vi "Actor Core.vi"(8 "error in":errorcluster, 11 "Interlock in":refnum<class "Interlock.lvclass">) -> (0 "error out":errorcluster, 3 "Actor out":refnum<class "Actor.lvclass">)   [LabVIEW 2015, in "Interlocks.lvlib" / "Interlock.lvclass"]
doc: "(<B>Filename</B>: Actor Framework.lvlib:Actor.lvclass:Actor Core.vi)\n\nReceives messages to the actor, reacts to them, and initiates any error handling that may shut the actor down.\n\nDescendant classes may override this VI to append parallel tasks for the actor to complete while it handles messages. Overrides use the Call Parent Method node."
uses:
  Interlock.lvclass
  <vilib>/ActorFramework/Actor/Actor.lvclass
  <vilib>/ActorFramework/Actor/Actor.lvclass/Actor.ctl
  <vilib>/ActorFramework/Message Enqueuer/Message Enqueuer.lvclass/Message Enqueuer.ctl
  <vilib>/ActorFramework/Message Enqueuer/Enqueue.vi
  <vilib>/ActorFramework/Message Enqueuer/Init from Existing Queue.vi
  <vilib>/ActorFramework/Message Priority Queue/Priority Enqueue.vi
  Interlock Messages/Invoke IL Action Msg/Invoke IL Action Msg.lvclass
  <vilib>/ActorFramework/Message Enqueuer/Message Enqueuer.lvclass
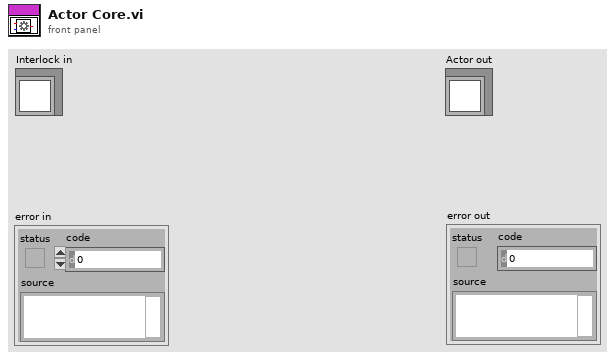
[diagram p1: front panel]
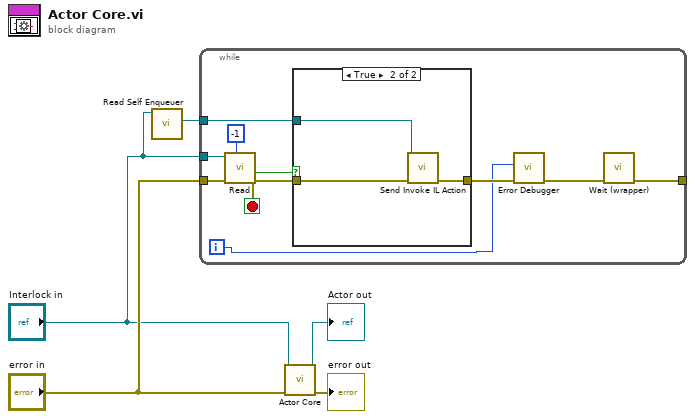
[diagram p0: block diagram]
diagram:
  n1 = call <vilib>:"Read Self Enqueuer.vi"("Actor"="Interlock in") -> ("Self Enqueuer"=w1:refnum<class "Message Enqueuer.lvclass">)  [unwired: 10 in]
  n2 = while {
    tunnel: "Interlock in" -> [w14]
    tunnel: "error in" -> [w13]
    tunnel: w1 -> [w10]
    tunnel: [w9] -> _
    i -> [w6]
    stop <- w11 stop-if-true
    n3 = call-dynamic "Read.vi"("timeout (100ms)"=-1, "error in (no error)"=w13, "Interlock in"=w14) -> ("error out"=w11:errorcluster, "Interlock out"=w12:bool)  [unwired: 4 in, 3 out]
    n4 = case shown="True" w12 {
      tunnel: w11 -> [w16 w19]
      tunnel: w10 -> [_ w18]
      tunnel: [w16 w17] -> w8
      frame False {
      }
      frame True {
        n5 = call "Send Invoke IL Action.vi"("error in (no error)"=w19, "Message Enqueuer"=w18) -> ("error out"=w17:errorcluster)  [unwired: 8 in, 1 out]
      }
    }
    n6 = call "Error Debugger.vi"("error in (no error)"=w8, "Numeric"=w6) -> ("error out"=w7:errorcluster)  [unwired: 9 in]
    n7 = call "Wait (wrapper).vi"("error in (no error)"=w7) -> ("error out"=w9:errorcluster)  [unwired: 10 in]
  }
  n8 = call-parent "Actor Core.vi"("error in"="error in", "Actor in"="Interlock in") -> ("error out"=→"error out":errorcluster, "Actor out"=→"Actor out":refnum<class "Actor.lvclass">)  [unwired: 8 in]
